vi "EOLerrorStringToInteger.vi"(9 "targetLength":i32, 11 "binaryString":string) -> (1 "\\nRemoved":i32, 3 "trimmedSelectiveReplaceData":i16[](array[numeric]))   [LabVIEW 2020]
uses:
  <vilib>/Analysis/NI_AALBase.lvlib
panel:
  out "\\r\\nFound":i32
  out "total\\r\\n":i32
  out "size(s) 3":i32 caption="Length"
  out "standard deviation 3":dbl caption="SD"
  out "standard deviation 2":dbl
  out "standard deviation":dbl
  out "size(s) 2":i32
  out "size(s)":i32
  out "retrievedData":i16[][](graph)
  # "WARNING- PROCESSING DATA WITH CUSTOM TRANSLATOR TO CORRECT EOL ERRORS"
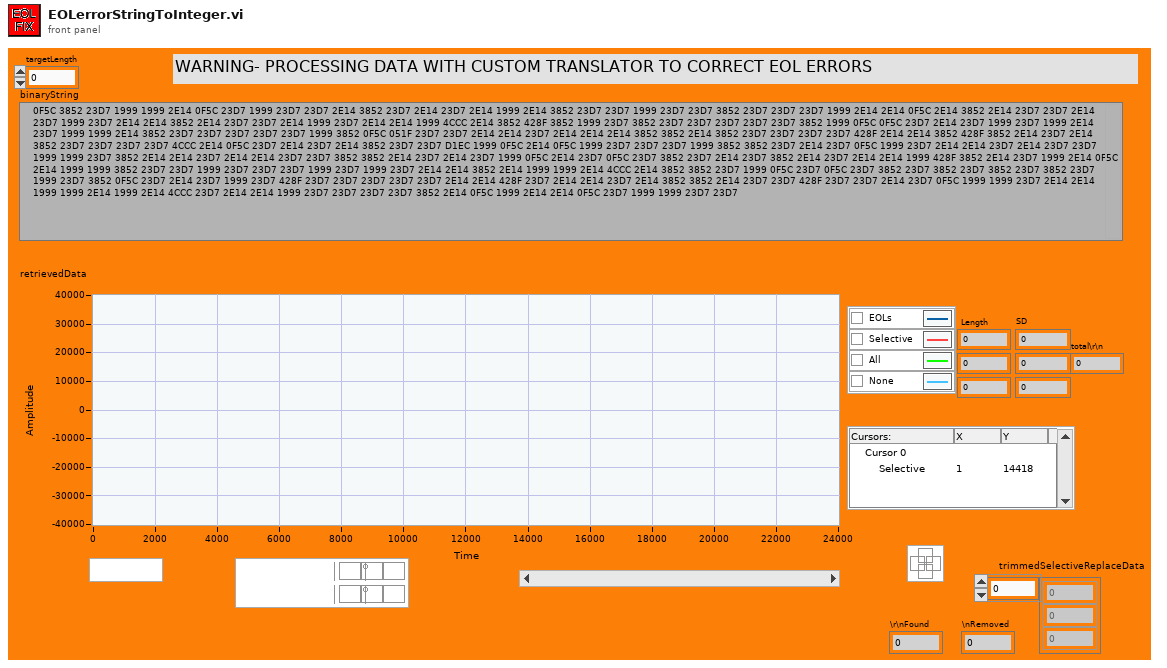
[diagram p1: front panel]
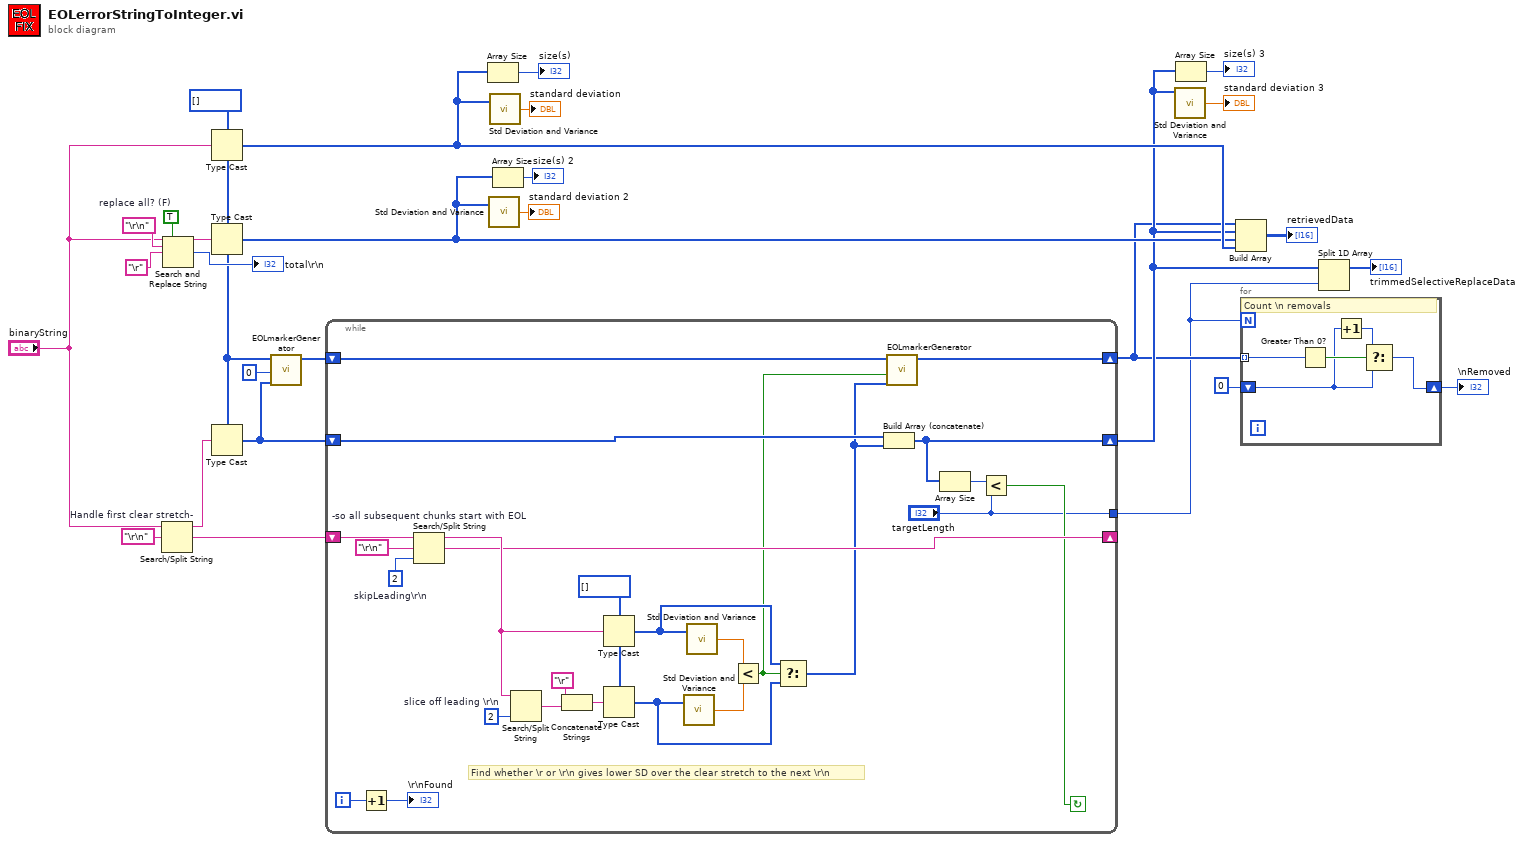
[diagram p0: block diagram]
diagram:
  w6 = i16[] [] ("Array - Numeric")
  w25 = TRUE  # replace all? (F)
  n1 = Search/Split String "Handle first clear stretch-"(string="binaryString", search string/char (-)="\r\n" ("search string")) -> (substring before match=w18:string, match + rest of string=w17:string)  [unwired: 1 in, 1 out]
  n2 = Search and Replace String(replace all?=w25, input string="binaryString", search string="\r\n", replace string="\r" ("replace string (\"\")")) -> (result string=w23:string, number of replacements=→"total\\r\\n":i32)  [unwired: 4 in, 2 out]
  n3 = Type Cast(type=w6, x="binaryString") -> (*(type *) &x=w13:i16[])
  n4 = Type Cast(type=w6, x=w23) -> (*(type *) &x=w12:i16[])
  n5 = Type Cast(type=w6, x=w18) -> (*(type *) &x=w7:i16[])
  n6 = call "EOLmarkerGenerator.vi"("chunk"=w7, "markerValue"=i16 0, "markerArrayIn"=w6) -> ("markerArrayOut"=w15:i16[])  [unwired: 8 in]
  n7 = while {
    shift-right: [w42] -> _
    shift-left: w17 -> [w46]
    shift-right: [w37] -> w11
    shift-left: w7 -> [w39]
    shift-right: [w30] -> w5
    shift-left: w15 -> [w31]
    tunnel: ["targetLength"] -> w1
    i -> [w34]
    stop <- w36 continue-if-true
    w44 = 2  # skipLeading\r\n
    w50 = 2  # slice off leading \r\n
    w51 = i16[] [] ("Array - Numeric")
    # "Find whether \\r or \\r\\n gives lower SD over the clear stretch to the next \\r\\n"
    n8 = Increment(x=w34) -> (x+1=→"\\r\\nFound":i32)
    n9 = Search/Split String "-so all subsequent chunks start with EOL"(string=w46, search string/char (-)="\r\n" ("search string"), offset (0)=w44) -> (substring before match=w43:string, match + rest of string=w42:string)  [unwired: 1 out]
    n10 = Search/Split String(string=w43, offset (0)=w50) -> (match + rest of string=w52:string)  [unwired: 1 in, 2 out]
    n11 = Concatenate Strings("\r" ("string"), w52) -> (w47:string)
    n12 = Type Cast(type=w51, x=w43) -> (*(type *) &x=w41:i16[])
    n13 = Type Cast(type=w51, x=w47) -> (*(type *) &x=w40:i16[])
    n14 = call <vilib>:"Std Deviation and Variance.vi"("X"=w40) -> ("standard deviation"=w48:dbl)  [unwired: 1 in, 2 out]
    n15 = call <vilib>:"Std Deviation and Variance.vi"("X"=w41) -> ("standard deviation"=w49:dbl)  [unwired: 1 in, 2 out]
    n16 = Less?(x=w49, y=w48) -> (x < y?=w38:bool)
    n17 = Select(t=w41, s=w38, f=w40) -> (s? t:f=w32:i16[])
    n18 = Build Array (concatenate)(w39, w32) -> (w37:i16[])
    n19 = call "EOLmarkerGenerator.vi"("chunk"=w32, "Polarity"=w38, "markerArrayIn"=w31) -> ("markerArrayOut"=w30:i16[])  [unwired: 8 in]
    n20 = Array Size(array=w37) -> (size(s)=w35:i32)
    n21 = Less?(x=w35, y="targetLength") -> (x < y?=w36:bool)
  }
  n22 = Array Size(array=w13) -> (size(s)=→"size(s)":i32)
  n23 = call <vilib>:"Std Deviation and Variance.vi"("X"=w12) -> ("standard deviation"=→"standard deviation 2":dbl)  [unwired: 1 in, 2 out]
  n24 = call <vilib>:"Std Deviation and Variance.vi"("X"=w13) -> ("standard deviation"=→"standard deviation":dbl)  [unwired: 1 in, 2 out]
  n25 = Array Size(array=w12) -> (size(s)=→"size(s) 2":i32)
  n26 = call <vilib>:"Std Deviation and Variance.vi"("X"=w11) -> ("standard deviation"=→"standard deviation 3":dbl)  [unwired: 1 in, 2 out]
  n27 = Array Size(array=w11) -> (size(s)=→"size(s) 3":i32)
  n28 = Build Array(w5, w11, w12, w13) -> (→"retrievedData":i16[][])
  n29 = for {
    N: w1 -> [_]
    tunnel: w5 -> [w58] mode=indexing
    shift-right: [w54] -> w3
    shift-left: 0 -> [w56]
    # "Count \\n removals"
    n30 = Greater Than 0?(x=w58) -> (x > 0?=w57:bool)
    n31 = Increment(x=w56) -> (x+1=w55:i32)
    n32 = Select(t=w55, s=w57, f=w56) -> (s? t:f=w54:i32)
  }
  "\\nRemoved" <- w3
  n33 = Split 1D Array(array=w11, index=w1) -> (first subarray=→"trimmedSelectiveReplaceData":i16[])  [unwired: 1 out]
